vi "TestSampler.vi"() -> ()   [LabVIEW 2023, in "Zone.lvclass"]
uses:
  Zone.lvclass
  Field_class/Field.lvclass
panel:
  in  "Array":dbl[][](array[numeric])
  in  "OK Button":bool
  out "Intensity Graph":dbl[][](graph)
  in  "step":dbl=500.0
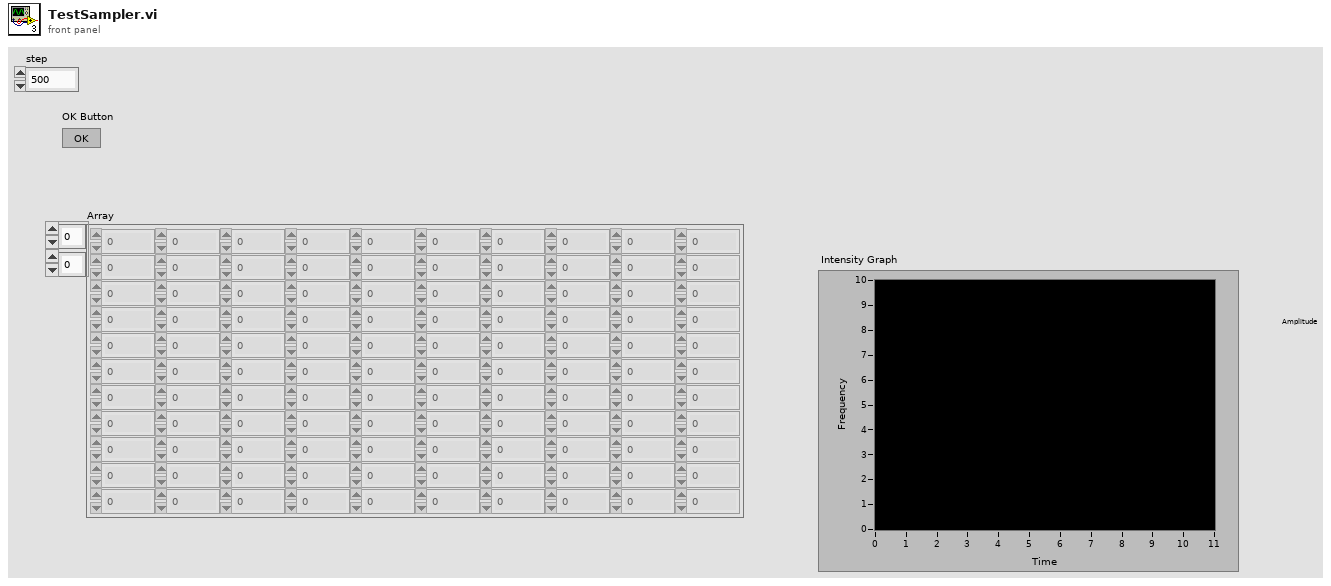
[diagram p1: front panel]
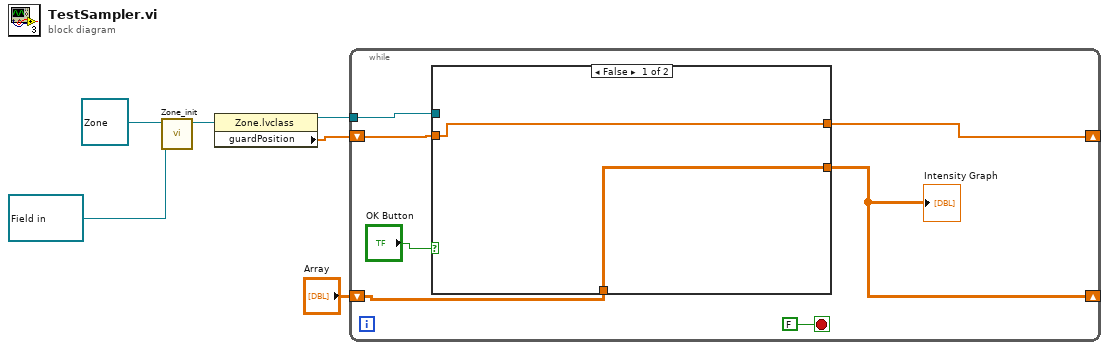
[diagram p0: block diagram]
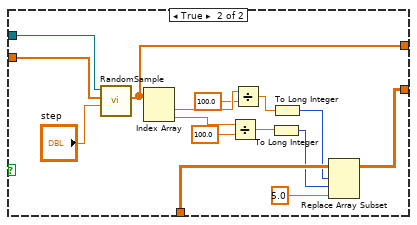
[diagram p2: hidden frame]
diagram:
  n1 = call "Zone_init.vi"("FieldDVR"=refnum<data-value> refnum, "Zone in"=refnum<class "Zone.lvclass"> refnum ("Zone.lvclass")) -> ("Zone out"=w4:refnum<class "Zone.lvclass">)  [unwired: 8 in, 1 out]
  n2 = property class="Zone.lvclass"(reference=w4) -> (reference out=w2:refnum<class "Zone.lvclass">, "guardPosition"=w3:dbl[])  [unwired: 1 in, 1 out]
  n3 = while {
    tunnel: w2 -> [w12]
    shift-right: [w8] -> _
    shift-left: "Array" -> [w10]
    shift-right: [w7] -> _
    shift-left: w3 -> [w13]
    stop <- FALSE stop-if-true
    n4 = case shown="False" "OK Button" {
      tunnel: w13 -> [w14 w29]
      tunnel: w12 -> [_ w28]
      tunnel: [w15 w23] -> w8
      tunnel: w10 -> [w15 w27]
      tunnel: [w14 w16] -> w7
      frame False {
      }
      frame True {
        n5 = call "RandomSample.vi"("step"="step", "basePoint"=w29, "object in"=w28) -> ("randomPoint"=w16:dbl[])  [unwired: 6 in, 2 out]
        n6 = Index Array(array=w16) -> (element #1=w22:dbl, element #2=w20:dbl)  [unwired: 2 in]
        n7 = Divide(x=w20, y=100.0) -> (x/y=w21:dbl)
        n8 = Divide(x=w22, y=100.0) -> (x/y=w17:dbl)
        n9 = To Long Integer(number=w21) -> (32bit integer=w25:i32)
        n10 = To Long Integer(number=w17) -> (32bit integer=w26:i32)
        n11 = Replace Array Subset(array=w27, new element=5.0 ("new element/subarray"), index (row)=w26, index (col)=w25) -> (w23:dbl[][])
      }
    }
    "Intensity Graph" <- w8
  }
